vi "Read Count Measurement.vi"   [LabVIEW 2010, in "Agilent 2000 3000 X-Series.lvlib"]
doc: "Reads count measurement results."
uses:
  <instrlib>/Agilent 2000 3000 X-Series/Agilent 2000 3000 X-Series.lvlib
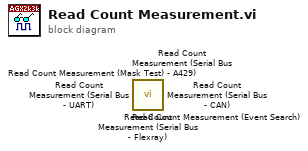
[diagram p0: block diagram]
diagram:
  n1 = call <instrlib>:"Read Count Measurement (Serial Bus - Flexray).vi"() -> ()  [unwired: 7 in, 5 out]
  n2 = call <instrlib>:"Read Count Measurement (Serial Bus - A429).vi"() -> ()  [unwired: 8 in, 4 out]
  n3 = call <instrlib>:"Read Count Measurement (Serial Bus - UART).vi"() -> ()  [unwired: 7 in, 5 out]
  n4 = call <instrlib>:"Read Count Measurement (Serial Bus - CAN).vi"() -> ()  [unwired: 6 in, 6 out]
  n5 = call <instrlib>:"Read Count Measurement (Mask Test).vi"() -> ()  [unwired: 7 in, 5 out]
  n6 = call <instrlib>:"Read Count Measurement (Event Search).vi"() -> ()  [unwired: 9 in, 3 out]
